vi "Display path SubVi.vi"(2 "Array":T1(array[cluster]), 3 "Combo Box":string(combo)) -> (0 "Total Time":dbl, 1 "Total Path":dbl)   [LabVIEW 2017]
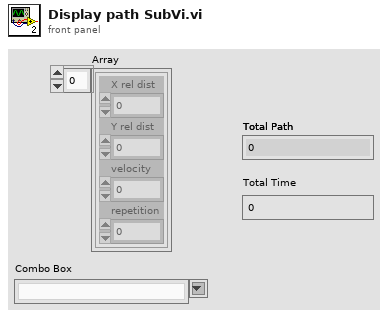
[diagram p1: front panel]
types:
  T1 = cluster{"X rel dist":dbl, "Y rel dist":dbl, "velocity":dbl, "repetition":u32}[]
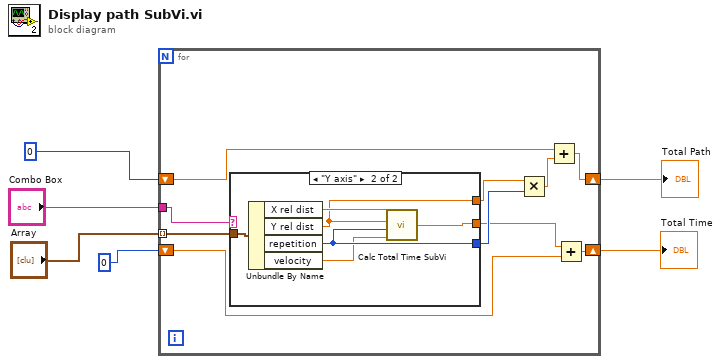
[diagram p0: block diagram]
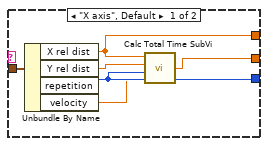
[diagram p2: hidden frame]
diagram:
  n1 = for {
    shift-right: [w13] -> w5
    shift-left: 0 -> [w16]
    tunnel: "Array" -> [w14] mode=indexing
    tunnel: "Combo Box" -> [w12]
    shift-right: [w7] -> w1
    shift-left: 0 -> [w8]
    n2 = case shown="\"Y axis\"" w12 {
      tunnel: [w21 w26] -> w11
      tunnel: [w19 w25] -> w10
      tunnel: w14 -> [w22 w28]
      tunnel: [w17 w23] -> w9
      frame "X axis", Default {
        n3 = Unbundle By Name(w22) -> ("X rel dist"=w21:dbl, "Y rel dist"=w20:dbl, "repetition"=w19:u32, "velocity"=w18:dbl)
        n4 = call "Calc Total Time SubVi.vi"("Vel"=w18, "rep"=w19, "Y length"=w20, "X length"=w21) -> ("Total Time"=w17:dbl)
      }
      frame "Y axis" {
        n5 = Unbundle By Name(w28) -> ("X rel dist"=w27:dbl, "Y rel dist"=w26:dbl, "repetition"=w25:u32, "velocity"=w24:dbl)
        n6 = call "Calc Total Time SubVi.vi"("Vel"=w24, "rep"=w25, "Y length"=w26, "X length"=w27) -> ("Total Time"=w23:dbl)
      }
    }
    n7 = Multiply(x=w11, y=w10) -> (x*y=w15:dbl)
    n8 = Add(x=w16, y=w15) -> (x+y=w13:dbl)
    n9 = Add(x=w9, y=w8) -> (x+y=w7:dbl)
  }
  "Total Path" <- w5
  "Total Time" <- w1
